vi "Window-8-bit Export type dialogue.vi"() -> (1 "Cancelled":bool, 3 "Export type":T1(ring))   [LabVIEW 2017]
uses:
  Global Variables/General Globals.vi
panel:
  in  "Export type":T1(ring)=enum."Export from cursors selection"
  in  "Cancel":bool
  in  "Export":bool
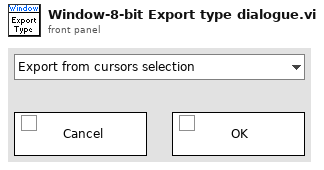
[diagram p1: front panel]
types:
  T1 = enum16{"Export from full dataset", "Export from cursors selection"}
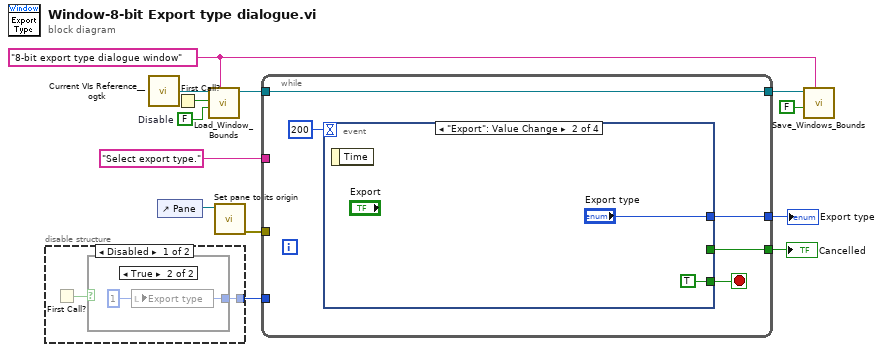
[diagram p0: block diagram]
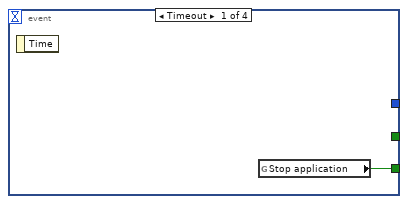
[diagram p4: hidden frame]
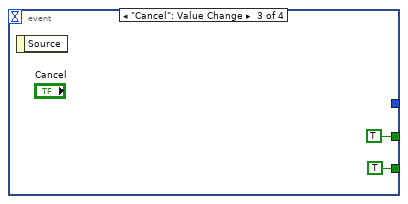
[diagram p5: hidden frame]
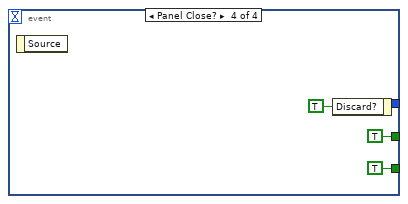
[diagram p6: hidden frame]
diagram:
  w9 = FALSE  # Disable
  w8 = "8-bit export type dialogue window" ("Window Name (i.e. Key)")
  n1 = disable-structure shown="Disabled" {
    disable-tunnel: [w14 _] -> w1
    frame Disabled {
      n2 = First Call?() -> (First Call?: T/F=w15:bool)
      n3 = case shown="True" w15 {
        tunnel: [_ w16] -> w14
        frame False {
        }
        frame True {
          w16 = 1
          n4 = local write "Export type"(w16) -> ()
        }
      }
    }
    frame Enabled {
    }
  }
  n5 = call <userlib>:"Current VIs Reference__ogtk.vi"() -> ("Current VI's reference"=w11:refnum<vi>)  [unwired: 5 in]
  n6 = control-ref of="Pane"() -> (w13:refnum<vi>)
  n7 = First Call?() -> (First Call?: T/F=w10:bool)
  n8 = call "Load_Window_Bounds.vi"("Window Name (i.e. Key)"=w8, "Disable"=w9, "First Call"=w10, "Window VI's Ref"=w11) -> ("reference out"=w5:refnum<vi>)  [unwired: 4 in, 3 out]
  n9 = call <userlib>:"Set pane to its origin.vi"("Pane Reference"=w13) -> ("error out (no error)"=w12:errorcluster)  [unwired: 9 in, 1 out]
  n10 = while {
    tunnel: w12 -> [_]
    tunnel: w5 -> [w19]
    tunnel: [w19] -> w6
    tunnel: "Select export type." ("Message display") -> [_]
    tunnel: [w18] -> w3
    tunnel: [w17] -> w2
    tunnel: w1 -> [_]
    stop <- w21 stop-if-true
    n11 = event shown="[1] \"Export\": Value Change" {
      selector: _ -> [_ _ _ _]
      dyn-events: _ -> [_ _ _ _]
      timeout: 200 -> [_ _ _ _]
      tunnel: [w22 TRUE TRUE TRUE] -> w21
      tunnel: [_ _ TRUE TRUE] -> w18
      tunnel: [_ "Export type" _ _] -> w17
      event Timeout {
        n12 = event-data() -> ()  [unwired: 1 in, 1 out]
        n13 = global read "General Globals.vi" "Stop application"() -> (w22:bool)
      }
      event "Export": Value Change {
        n14 = event-data() -> ()  [unwired: 1 in, 1 out]
      }
      event "Cancel": Value Change {
        n15 = event-data() -> ()  [unwired: 1 in, 1 out]
      }
      event Panel Close? {
        n16 = event-data() -> ()  [unwired: 1 in, 1 out]
        n17 = event-data("Discard?"=TRUE) -> ()  [unwired: 1 in, 1 out]
      }
    }
  }
  "Cancelled" <- w3
  "Export type" <- w2
  n18 = call "Save_Windows_Bounds.vi"("Window Name (i.e. Key)"=w8, "Front Panel Window:Open"=FALSE, "Window VI's Ref"=w6) -> ()  [unwired: 8 in, 1 out]
